vi "main.vi"(8 "error in (no error)":errorcluster, 11 "splash_screen in":refnum<class "splash_screen.lvclass">) -> (0 "error out":errorcluster, 3 "splash_screen out":refnum<class "splash_screen.lvclass">)   [LabVIEW 2020, in "splash_screen.lvclass"]
uses:
  splash_screen.lvclass
  <vilib>/sklein/WebView2/Webview2 Control/WebView2 Control.xctl
panel:
  in  "WebView2 Control":string(xcontrol)
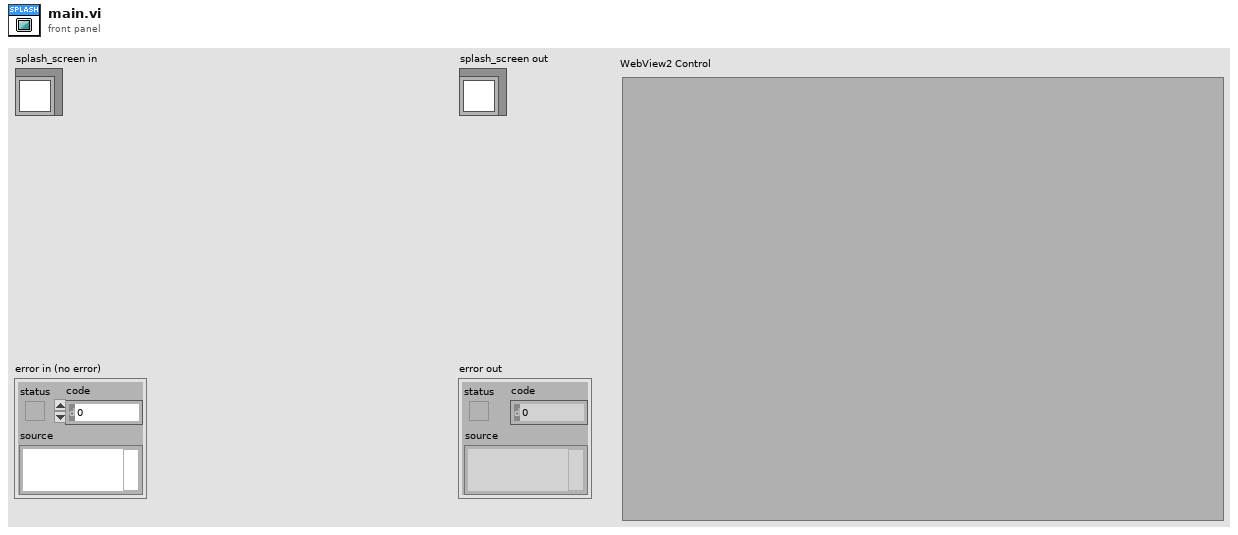
[diagram p1: front panel]
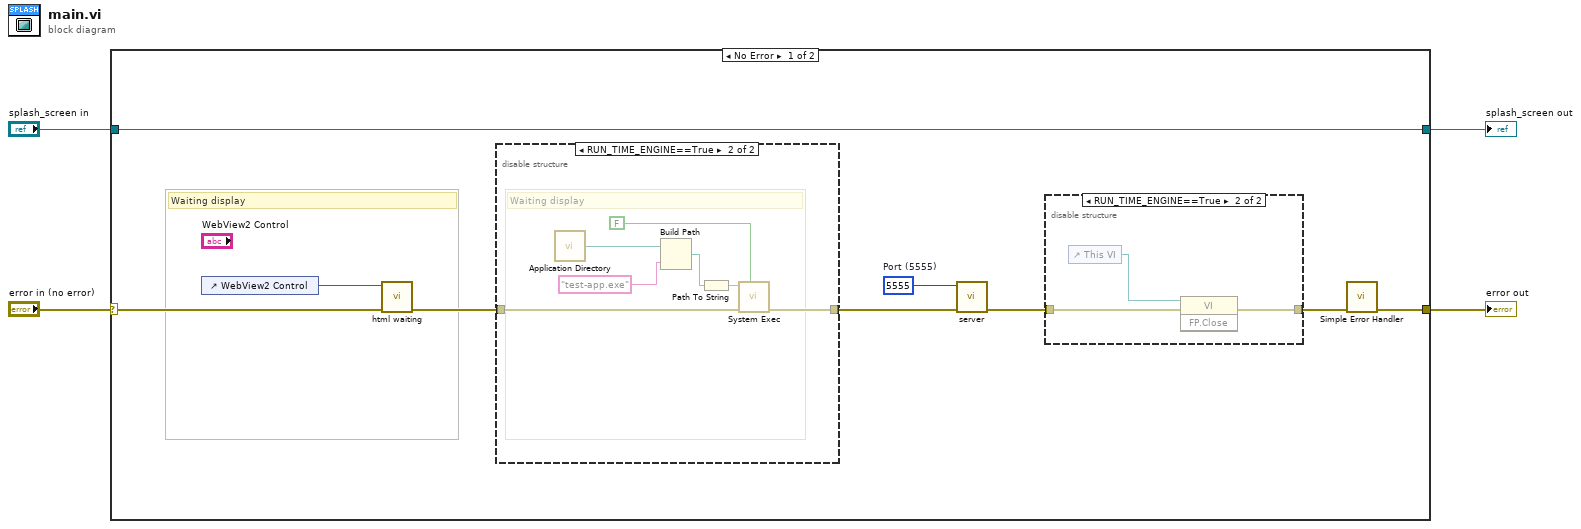
[diagram p0: block diagram]
diagram:
  n1 = case shown="No Error" "error in (no error)" {
    selector: "error in (no error)" -> [w7 w26]
    tunnel: [w8 w26] -> w3
    tunnel: [w13 w25] -> w1
    tunnel: "splash_screen in" -> [w13 w25]
    frame No Error {
      w12 = 5555  # Port (5555)
      # "Waiting display"
      n2 = control-ref of="WebView2 Control"() -> (w9:refnum<vi>)
      n3 = call "html waiting.vi"("error in (no error)"=w7, "WebView2 Control"=w9) -> ("error out"=w6:errorcluster)  [unwired: 9 in]
      n4 = disable-structure shown="RUN_TIME_ENGINE==True" {
        disable-tunnel: w6 -> [w17 w24]
        disable-tunnel: [w17 w19] -> w5
        frame condition #0 (active) {
        }
        frame condition #1 {
          # "Waiting display"
          n5 = call <vilib>:"Application Directory.vi"() -> ("Application Directory"=w23:path)
          n6 = Build Path(base path=w23, name or relative path="test-app.exe" ("command line")) -> (appended path=w21:path)
          n7 = Path To String(path=w21) -> (string=w20:string)
          n8 = call <vilib>:"System Exec.vi"("wait until completion? (T)"=FALSE, "error in (no error)"=w24, "command line"=w20) -> ("error out"=w19:errorcluster)  [unwired: 5 in, 3 out]
        }
      }
      n9 = call "server.vi"("error in (no error)"=w5, "Port (5555)"=w12) -> ("error out"=w10:errorcluster)  [unwired: 9 in]
      n10 = disable-structure shown="RUN_TIME_ENGINE==True" {
        disable-tunnel: [_ w15] -> w11
        disable-tunnel: w10 -> [_ w16]
        frame condition #0 (active) {
        }
        frame condition #1 {
          n11 = control-ref of="This VI"() -> (w14:refnum<vi>)
          n12 = invoke class="VI" method="FP.Close"(reference=w14, error in=w16) -> (error out=w15:errorcluster)  [unwired: 1 in, 2 out]
        }
      }
      n13 = call <vilib>:"Simple Error Handler.vi"("error in (no error)"=w11) -> ("error out"=w8:errorcluster)  [unwired: 4 in, 4 out]
    }
    frame Error {
    }
  }
  "error out" <- w3
  "splash_screen out" <- w1
